vi "Create Statement from CSV.vi"(8 "error in (no error)":errorcluster, 11 "CSV Entries":string[](array[string])) -> (0 "error out":errorcluster, 3 "Credit Statement out":refnum<class "Credit Statement.lvclass">)   [LabVIEW 2018, in "Credit Statement.lvclass"]
uses:
  Credit Statement.lvclass
  C:/GitRepos/Filthy-Lucre-Budgetizer/source/support/classes/Statement/Statement.lvclass
  Credit Record/Credit Transaction.lvclass
  C:/GitRepos/Filthy-Lucre-Budgetizer/source/support/classes/Transaction/Transaction.lvclass
  Statement/Statement.lvclass
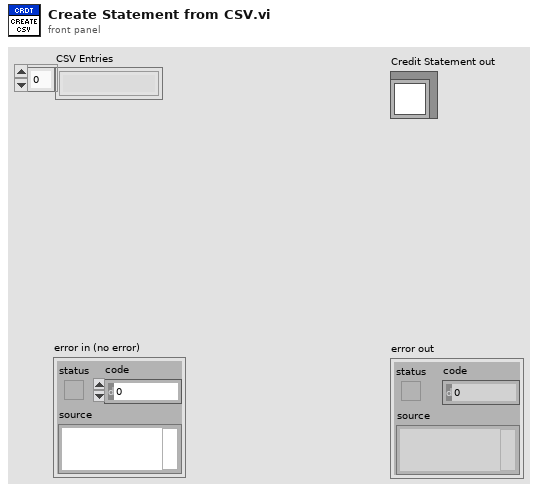
[diagram p1: front panel]
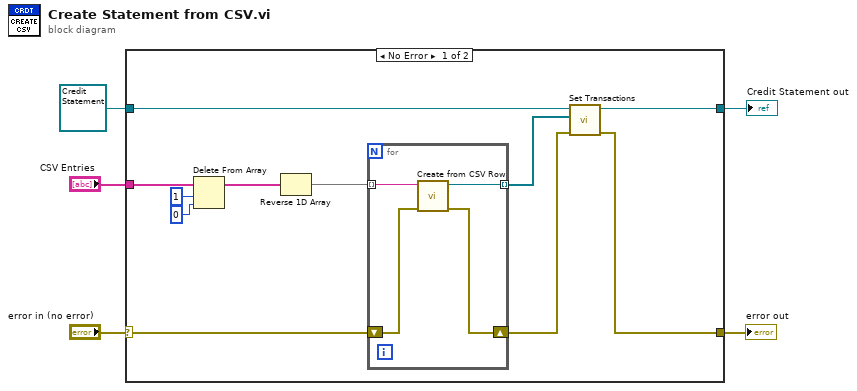
[diagram p0: block diagram]
diagram:
  n1 = case shown="No Error" "error in (no error)" {
    selector: "error in (no error)" -> [w16 w22]
    tunnel: [w6 w22] -> w4
    tunnel: [w9 w21] -> w2
    tunnel: refnum<class "Credit Statement.lvclass"> refnum ("Credit Statement.lvclass") -> [w10 w21]
    tunnel: "CSV Entries" -> [w13 _]
    frame No Error {
      n2 = Delete From Array(array=w13, length=1, index=0) -> (array with subset deleted=w12:string[])  [unwired: 1 out]
      n3 = Reverse 1D Array(array=w12) -> (reversed array=w11:string[])
      n4 = for {
        shift-right: [w18] -> w7
        shift-left: w16 -> [w19]
        tunnel: w11 -> [w20] mode=indexing
        tunnel: [w17] -> w8 mode=indexing
        n5 = call "Create from CSV Row.vi"("error in (no error)"=w19, "CSV Row"=w20) -> ("error out"=w18:errorcluster, "Credit Record out"=w17:refnum<class "Credit Transaction.lvclass">)  [unwired: 8 in]
      }
      n6 = call "Set Transactions.vi"("error in (no error)"=w7, "Transactions"=w8, "Statement in"=w10) -> ("error out"=w6:errorcluster, "Statement out"=w9:refnum<class "Credit Statement.lvclass">)  [unwired: 7 in]
    }
    frame Error {
    }
  }
  "error out" <- w4
  "Credit Statement out" <- w2
